vi "Parse-String-to-U8.vi"() -> ()   [LabVIEW 2017]
uses:
  <userlib>/_OpenG.lib/string/string.llb/Trim Whitespace (String)__ogtk.vi
panel:
  out "Ethernet Frame\n(u8 [])":u32[](array[numeric]) format="%.0x"
  in  "String":string
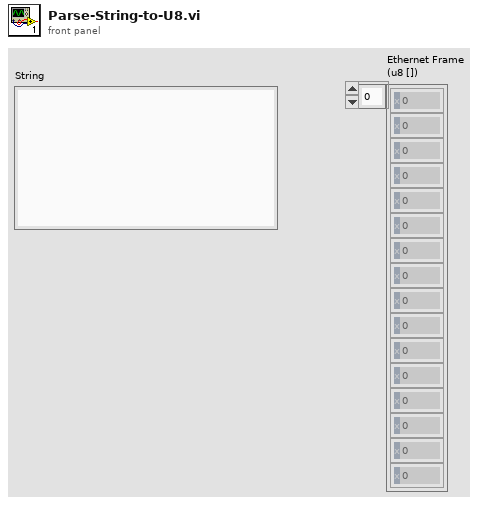
[diagram p1: front panel]
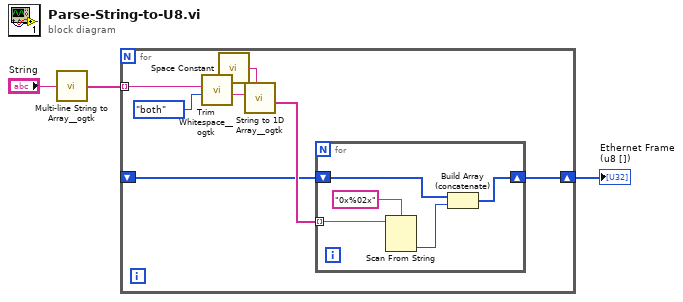
[diagram p0: block diagram]
diagram:
  n1 = call <userlib>:"Multi-line String to Array__ogtk.vi"("string"="String") -> ("lines"=w2:string[])
  n2 = for {
    tunnel: w2 -> [w10] mode=indexing
    shift-right: [w5] -> w1
    shift-left: _ -> [w4]
    n3 = call-poly <userlib>:"Trim Whitespace__ogtk.vi"("Remove (leading and trailing)"=enum16{"leading", "trailing", "both"}."both", "String in"=w10) -> ("String out"=w7:string)  [unwired: 5 in]
    n4 = call <vilib>:"Space Constant.vi"() -> ("String"=w8:string)
    n5 = call <userlib>:"String to 1D Array__ogtk.vi"("delimiter (Tab)"=w8, "string"=w7) -> ("Array of Strings"=w6:string[])  [unwired: 9 in]
    n6 = for {
      tunnel: w6 -> [w15] mode=indexing
      shift-right: [w12] -> w5
      shift-left: w4 -> [w11]
      n7 = Scan From String(format string="0x%02x", input string=w15) -> (output 1=w13:u32)  [unwired: 3 in, 3 out]
      n8 = Build Array (concatenate)(w11, w13) -> (w12:u32[])
    }
  }
  "Ethernet Frame\n(u8 [])" <- w1
